vi "update_key_state.vi"(9 "Array in":bool[](array[boolean]), 10 "down?":bool, 11 "ScanCode":i16) -> (3 "Array out":bool[](array[boolean]))   [LabVIEW 2025]
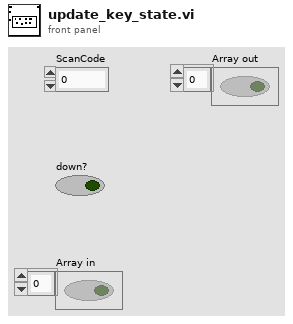
[diagram p1: front panel]
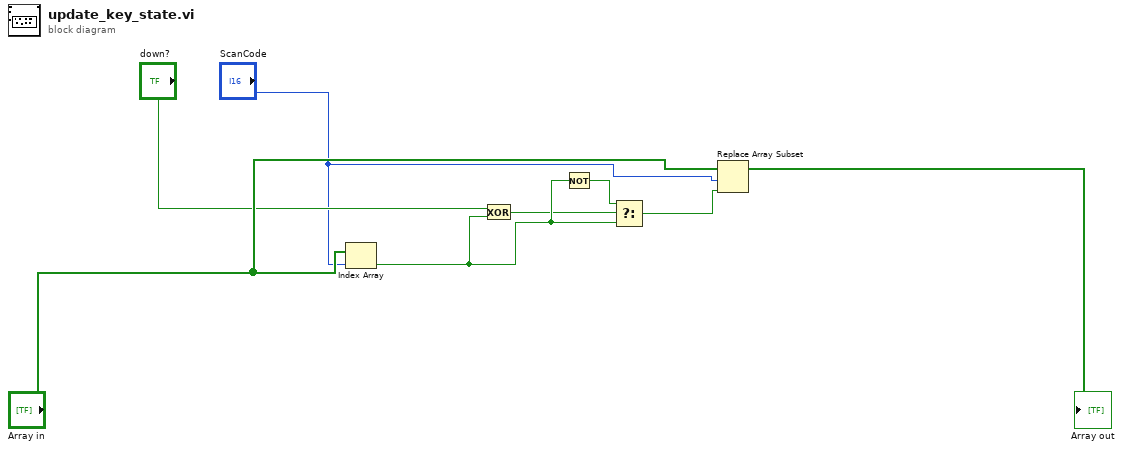
[diagram p0: block diagram]
diagram:
  n1 = Index Array(array="Array in", index="ScanCode") -> (element=w2:bool)
  n2 = Exclusive Or(1:w2, 2:"down?") -> (0:w1:bool)
  n3 = Not(x=w2) -> (.not. x?=w3:bool)
  n4 = Select(t=w3, s=w1, f=w2) -> (s? t:f=w4:bool)
  n5 = Replace Array Subset(array="Array in", new element=w4, index="ScanCode") -> (→"Array out":bool[])
